vi "Raw_input_to_sorted.vi"(10 "Input Array":dbl[](array[numeric])) -> (3 "Array Out":dbl[](array[numeric]))   [LabVIEW 2016]
doc: "This SubVI takes in Raw Serial Data and sorts it according to its adress"
panel:
  out "date string":string
  out "time string":string
  in  "New array":dbl[](array[numeric])=[0.0, 0.0, 0.0, 0.0, 0.0, 0.0, 0.0, 0.0, 0.0, 0.0, 0.0, 0.0, 0.0, 0.0, 0.0, 0.0, 0.0, 0.0, 0.0, 0.0, 0.0, 0.0, 0.0, 0.0, 0.0, 0.0, 0.0, 0.0, 0.0, 0.0, 0.0, 0.0, 0.0, 0.0, 0.0, 0.0, 0.0, 0.0, 0.0]
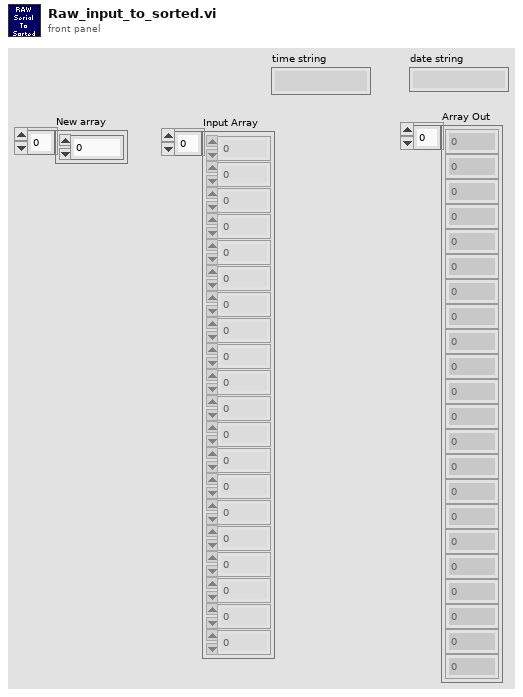
[diagram p1: front panel]
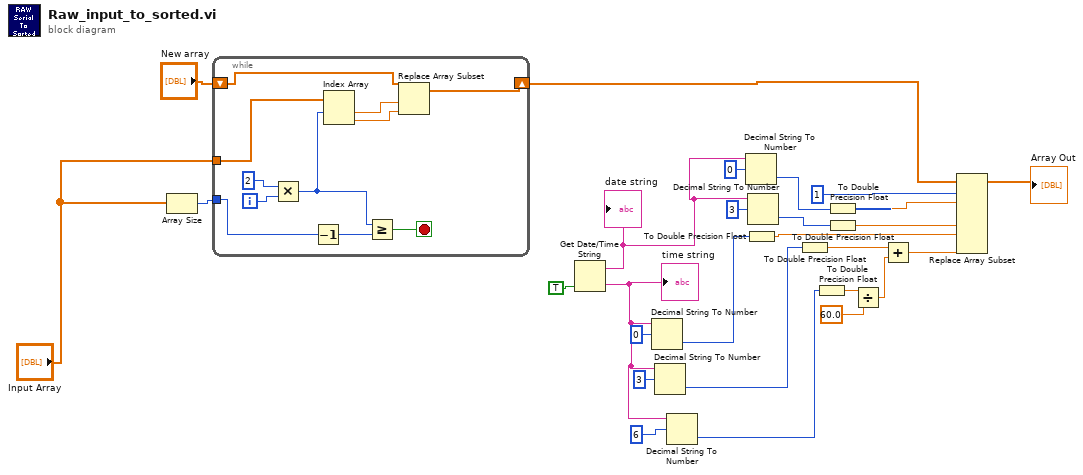
[diagram p0: block diagram]
diagram:
  n1 = Array Size(array="Input Array") -> (size(s)=w26:i32)
  n2 = while {
    tunnel: "Input Array" -> [w38]
    tunnel: w26 -> [w33]
    shift-right: [w28] -> w24
    shift-left: "New array" -> [w29]
    i -> [w35]
    stop <- w30 stop-if-true
    n3 = Multiply(x=2, y=w35) -> (x*y=w31:i32)
    n4 = Decrement(x=w33) -> (x-1=w32:i32)
    n5 = Index Array(array=w38, index #1=w31) -> (element #1=w37:dbl, element #2=w36:dbl)  [unwired: 1 in]
    n6 = Greater Or Equal?(x=w31, y=w32) -> (x >= y?=w30:bool)
    n7 = Replace Array Subset(array=w29, new element=w36, index=w37) -> (w28:dbl[])
  }
  n8 = Get Date/Time String(want seconds? (F)=TRUE) -> (date string=w7:string, time string=w19:string)  [unwired: 2 in]
  "time string" <- w19
  "date string" <- w7
  n9 = Decimal String To Number(string=w19, offset=0) -> (number=w16:i32)  [unwired: 1 in, 1 out]
  n10 = Decimal String To Number(string=w19, offset=3) -> (number=w15:i32)  [unwired: 1 in, 1 out]
  n11 = Decimal String To Number(string=w19, offset=6) -> (number=w14:i32)  [unwired: 1 in, 1 out]
  n12 = Decimal String To Number(string=w7, offset=0) -> (number=w3:i32)  [unwired: 1 in, 1 out]
  n13 = To Double Precision Float(number=w16) -> (double precision float=w9:dbl)
  n14 = Decimal String To Number(string=w7, offset=3) -> (number=w4:i32)  [unwired: 1 in, 1 out]
  n15 = To Double Precision Float(number=w15) -> (double precision float=w11:dbl)
  n16 = To Double Precision Float(number=w14) -> (double precision float=w13:dbl)
  n17 = To Double Precision Float(number=w3) -> (double precision float=w2:dbl)
  n18 = To Double Precision Float(number=w4) -> (double precision float=w1:dbl)
  n19 = Divide(x=w13, y=60.0) -> (x/y=w10:dbl)
  n20 = Add(x=w11, y=w10) -> (x+y=w8:dbl)
  n21 = Replace Array Subset(array=w24, new element #1=w2, index #1=1 ("index"), new element #2=w1, new element #3=w9, new element #4=w8) -> (→"Array Out":dbl[])  [unwired: 3 in]
